vi "calculate linear fit.vi"(8 "error in (no error)":errorcluster, 11 "Autofocus in":refnum<class "Autofocus.lvclass">) -> (0 "error out":errorcluster, 3 "Autofocus out":refnum<class "Autofocus.lvclass">)   [LabVIEW 2012, in "Autofocus.lvclass"]
uses:
  Autofocus.lvclass
  <vilib>/Analysis/6fits.llb/Curve Fitting Criteria.ctl
  Autofocus.lvclass/Autofocus.ctl
  <vilib>/Analysis/NI_AALPro.lvlib
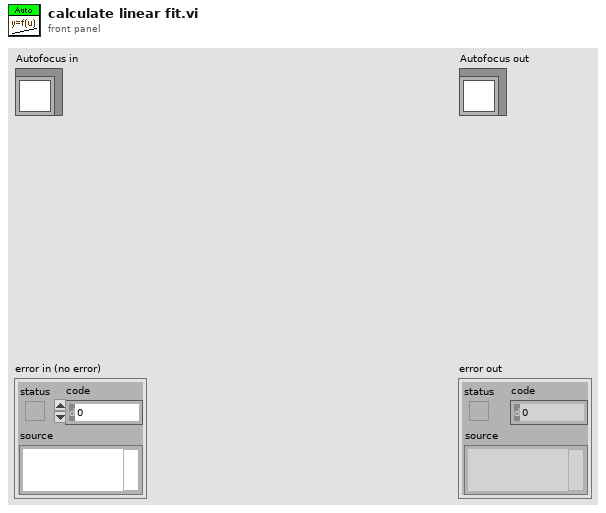
[diagram p1: front panel]
types:
  T1 = typedef "NI_AALPro.lvlib/Curve Fitting Criteria.ctl" = u16
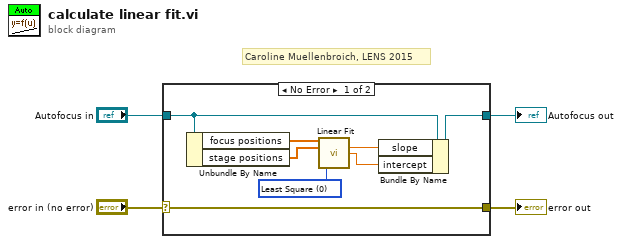
[diagram p0: block diagram]
diagram:
  # "Caroline Muellenbroich, LENS 2015"
  n1 = case shown="No Error" "error in (no error)" {
    selector: "error in (no error)" -> [w12 w14]
    tunnel: [w12 w14] -> w3
    tunnel: "Autofocus in" -> [w7 w13]
    tunnel: [w10 w13] -> w1
    frame No Error {
      w11 = T1 0 items=["Least Square", "Least Absolute Residual", "Bisquare"] ("method")
      n2 = Unbundle By Name(w7) -> ("focus positions"=w6:dbl[], "stage positions"=w5:dbl[])
      n3 = call <vilib>:"Linear Fit.vi"("Y"=w6, "X"=w5, "method"=w11) -> ("slope"=w9:dbl, "intercept"=w8:dbl)  [unwired: 8 in, 3 out]
      n4 = Bundle By Name(cluster=w7, "slope"=w9, "intercept"=w8) -> (w10:refnum<class "Autofocus.lvclass">)
    }
    frame Error {
    }
  }
  "error out" <- w3
  "Autofocus out" <- w1
